vi "publishTelemetryHardpointStatus.vi"(8 "error in (no error)":errorcluster, 11 "Model in":refnum<class "Model.lvclass">) -> (0 "error out":errorcluster, 3 "Model out":refnum<class "Model.lvclass">)   [LabVIEW 2016, in "Model.lvclass"]
uses:
  Model.lvclass
  Model.lvclass/Model.ctl
  Publisher/Publisher.lvclass
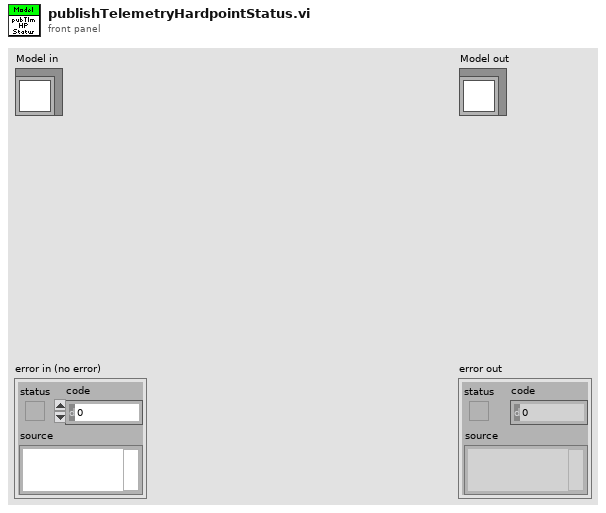
[diagram p1: front panel]
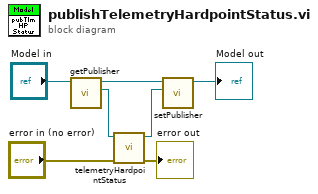
[diagram p0: block diagram]
diagram:
  n1 = call "getPublisher.vi"("Model in"="Model in") -> ("Publisher"=w5:refnum<class "Publisher.lvclass">, "Model out"=w4:refnum<class "Model.lvclass">)  [unwired: 9 in]
  n2 = call "telemetryHardpointStatus.vi"("error in (no error)"="error in (no error)", "Publisher in"=w5) -> ("error out"=→"error out":errorcluster, "Publisher out"=w3:refnum<class "Publisher.lvclass">)  [unwired: 8 in]
  n3 = call "setPublisher.vi"("Publisher"=w3, "Model in"=w4) -> ("Model out"=→"Model out":refnum<class "Model.lvclass">)  [unwired: 9 in]
